vi "smff_TimeInterpDouble_GetTimeForValue.vi"(9 "ValueToFind":dbl, 11 "TimeInterpDouble":T1) -> (1 "ValueFound":bool, 3 "TimeStamp":dbl)   [LabVIEW 2019]
doc: "Sample the buffer at the given time.\n\nInputs:\n - TimeInterpDouble -- Input data cluster\n - TimeStamp -- Time at which to sample (seconds)\n\nOutputs\n - OutputDouble -- Sampled Double. This is an exact value if there is a sample in the buffer at this time. Otherwise the value is interpolated. \n - IsPresent -- Returns TRUE if the buffer contains data as far back as TimeStamp."
uses:
  <vilib>/Rock Robotics/WPI/ThirdParty/JAS_Junk/TrajLib/TypeDef/TIME_INTERPOLATABLE_DOUBLE.ctl
  <vilib>/Rock Robotics/WPI/ThirdParty/JAS_Junk/TrajLib/MathUtil_Clamp.vi
  <vilib>/Rock Robotics/WPI/ThirdParty/JAS_Junk/TrajLib/Trajectory_Library.lvlib
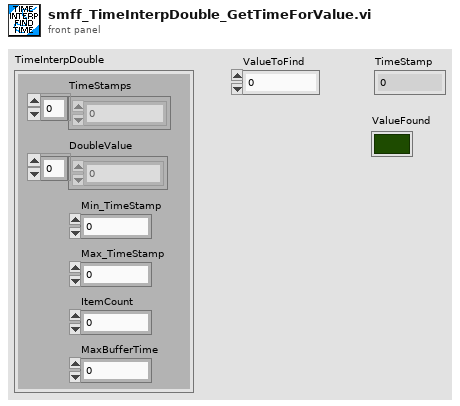
[diagram p1: front panel]
types:
  T1 = typedef "Trajectory_Library.lvlib/TIME_INTERPOLATABLE_DOUBLE.ctl" = cluster{"TimeStamps":dbl[], "DoubleValue":dbl[], "Min_TimeStamp":dbl, "Max_TimeStamp":dbl, "ItemCount":i32, "MaxBufferTime":dbl}
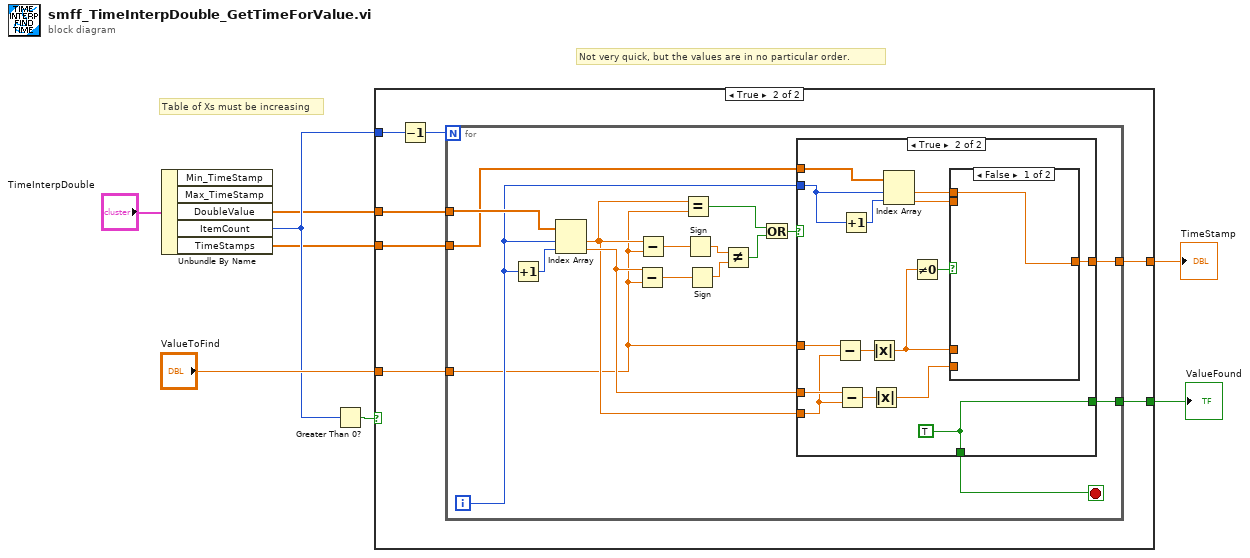
[diagram p0: block diagram]
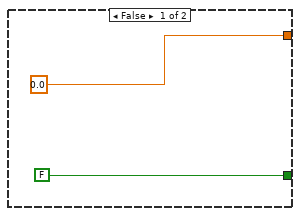
[diagram p2: hidden frame]
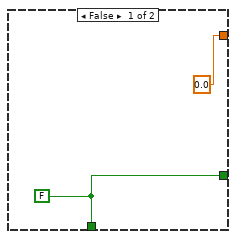
[diagram p3: hidden frame]
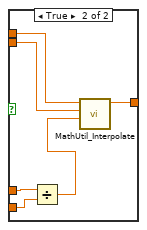
[diagram p4: hidden frame]
diagram:
  # "Not very quick, but the values are in no particular order."
  # "Table of Xs must be increasing"
  n1 = Unbundle By Name("TimeInterpDouble") -> ("DoubleValue"=w2:dbl[], "ItemCount"=w3:i32, "TimeStamps"=w1:dbl[])  [unwired: 2 out]
  n2 = Greater Than 0?(x=w3) -> (x > 0?=w5:bool)
  n3 = case shown="True" w5 {
    tunnel: "ValueToFind" -> [_ w13]
    tunnel: [0.0 w12] -> w7
    tunnel: [FALSE w11] -> w4
    tunnel: w3 -> [_ w16]
    tunnel: w2 -> [_ w15]
    tunnel: w1 -> [_ w14]
    frame False {
    }
    frame True {
      n4 = Decrement(x=w16) -> (x-1=w17:i32)
      n5 = for {
        N: w17 -> [_]
        tunnel: w15 -> [w33]
        tunnel: w14 -> [w25]
        tunnel: w13 -> [w21]
        tunnel: [w20] -> w12
        tunnel: [w18] -> w11
        i -> [w24]
        stop <- w19 stop-if-true
        n6 = Increment(x=w24) -> (x+1=w34:i32)
        n7 = Index Array(array=w33, index #1=w24, index #2=w34) -> (element #1=w22:dbl, element #2=w23:dbl)
        n8 = Subtract(x=w23, y=w21) -> (x-y=w31:dbl)
        n9 = Subtract(x=w22, y=w21) -> (x-y=w32:dbl)
        n10 = Equal?(x=w22, y=w21) -> (x = y?=w28:bool)
        n11 = Sign(1:w32) -> (0:w30:dbl)
        n12 = Sign(1:w31) -> (0:w29:dbl)
        n13 = Not Equal?(x=w30, y=w29) -> (x != y?=w27:bool)
        n14 = Or(x=w28, y=w27) -> (x .or. y?=w26:bool)
        n15 = case shown="True" w26 {
          tunnel: w25 -> [_ w50]
          tunnel: w24 -> [_ w49]
          tunnel: w23 -> [_ w45]
          tunnel: w22 -> [_ w42]
          tunnel: w21 -> [_ w43]
          tunnel: [0.0 ("InterpolatedValue") w41] -> w20
          tunnel: [w36 w40] -> w19
          tunnel: [w36 w40] -> w18
          frame False {
            w36 = FALSE
          }
          frame True {
            w40 = TRUE
            n16 = Subtract(x=w43, y=w42) -> (x-y=w44:dbl)
            n17 = Subtract(x=w45, y=w42) -> (x-y=w46:dbl)
            n18 = Increment(x=w49) -> (x+1=w51:i32)
            n19 = Absolute Value(x=w44) -> (abs(x)=w37:dbl)
            n20 = Absolute Value(x=w46) -> (abs(x)=w38:dbl)
            n21 = Index Array(array=w50, index #1=w49, index #2=w51) -> (element #1=w48:dbl, element #2=w47:dbl)
            n22 = Not Equal To 0?(x=w37) -> (x != 0?=w39:bool)
            n23 = case shown="False" w39 {
              tunnel: w48 -> [w52 w58]
              tunnel: w47 -> [_ w57]
              tunnel: [w52 w56] -> w41
              tunnel: w38 -> [_ w55]
              tunnel: w37 -> [_ w54]
              frame False {
              }
              frame True {
                n24 = Divide(x=w54, y=w55) -> (x/y=w53:dbl)
                n25 = call <vilib>:"MathUtil_Interpolate.vi"("T"=w53, "EndValue"=w57, "StartValue"=w58) -> ("InterpolatedValue"=w56:dbl)  [unwired: 8 in]
              }
            }
          }
        }
      }
    }
  }
  "TimeStamp" <- w7
  "ValueFound" <- w4
